vi "Test Nested Library Method.vi"(8 "error in (no error)":errorcluster, 11 "Library Nesting Library with Tests.lvlib:Nested Library with Test.lvlib:Test in Nested Library.lvclass":refnum<class "Test in Nested Library.lvclass">) -> (0 "error out":errorcluster, 3 "LUnit Test Case Out":refnum<class "Test in Nested Library.lvclass">)   [LabVIEW 2020, in "Library Nesting Library with Tests.lvlib" / "Nested Library with Test.lvlib" / "Test in Nested Library.lvclass"]
uses:
  Test in Nested Library.lvclass
  C:/git/astemes-lunit/source/LUnit Test Case.lvclass
  source/LUnit Test Case.lvclass/LUnit Test Case.ctl
  source/Core/LUnit Test Case/Private/Append Fail Result.vi
  source/Core/LUnit Test Case/Private/Run In UI.vi
  <vilib>/Utility/error.llb/Clear Errors.vi
  source/LUnit Test Case.lvclass
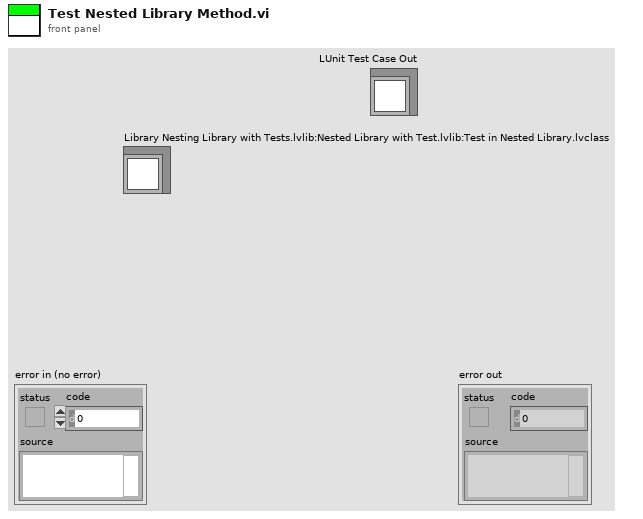
[diagram p1: front panel]
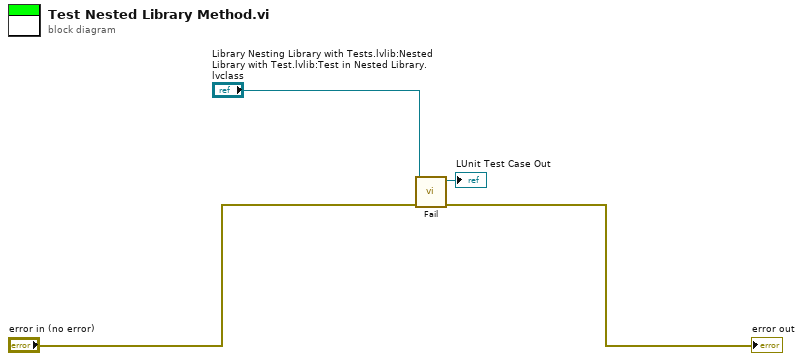
[diagram p0: block diagram]
diagram:
  n1 = call "Fail.vi"("error in (no error)"="error in (no error)", "LUnit Test Case In"="Library Nesting Library with Tests.lvlib:Nested Library with Test.lvlib:Test in Nested Library.lvclass") -> ("error out"=→"error out":errorcluster, "LUnit Test Case Out"=→"LUnit Test Case Out":refnum<class "Test in Nested Library.lvclass">)  [unwired: 8 in]
